vi "logarytmiczny.vi"(1 "Ilosc probek":u32, 2 "F min":dbl, 3 "F max":dbl) -> (0 "Array":dbl[](array[numeric]))   [LabVIEW 2021]
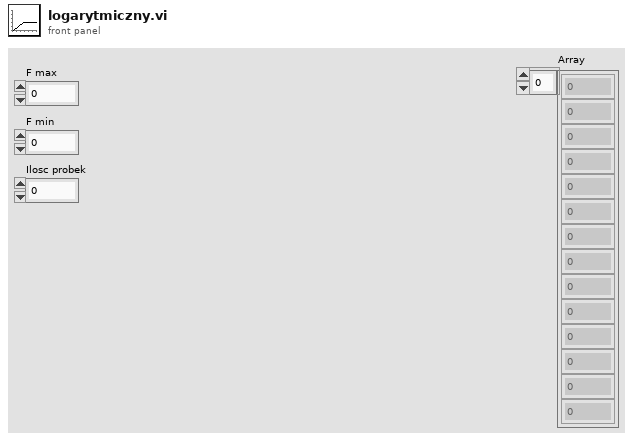
[diagram p1: front panel]
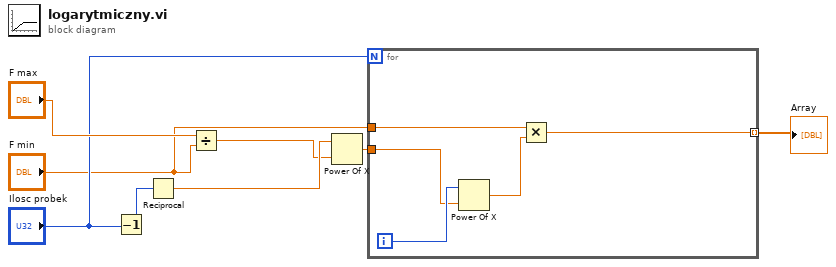
[diagram p0: block diagram]
diagram:
  n1 = Decrement(x="Ilosc probek") -> (x-1=w8:u32)
  n2 = Reciprocal(x=w8) -> (1/x=w7:dbl)
  n3 = Divide(x="F max", y="F min") -> (x/y=w5:dbl)
  n4 = Power Of X(1:w5, 2:w7) -> (0:w3:dbl)
  n5 = for {
    N: "Ilosc probek" -> [_]
    tunnel: w3 -> [w12]
    tunnel: "F min" -> [w11]
    tunnel: [w9] -> w1 mode=indexing
    i -> [w13]
    n6 = Power Of X(1:w12, 2:w13) -> (0:w10:dbl)
    n7 = Multiply(x=w11, y=w10) -> (x*y=w9:dbl)
  }
  "Array" <- w1
